vi "PupilFitEllipse.vi"(7 "Image Name":string="ellipse2", 8 "CR Ellipse":T2 {"Minor Axis"."Point 2"."Y" format="%.2f"; "Minor Axis"."Point 2"."X" format="%.2f"; "Minor Axis"."Point 1"."Y" format="%.2f"; "Minor Axis"."Point 1"."X" format="%.2f"; "Major Axis"."Point 2"."Y" format="%.2f"; "Major Axis"."Point 2"."X" format="%.2f"; "Major Axis"."Point 1"."Y" format="%.2f"; "Major Axis"."Point 1"."X" format="%.2f"; "Center"."Y" format="%.2f"; "Center"."X" format="%.2f"}, 9 "r":dbl=100.0, 10 "rough center":cluster{"Pos. X":i32, "Pos. Y":i32}, 11 "Image Src":T3) -> (0 "输出簇":T1, 1 "Image Out":T3, 2 "Valid Fit":bool, 3 "Ellipse 2":T2 {"Minor Axis"."Point 2"."Y" format="%.2f"; "Minor Axis"."Point 2"."X" format="%.2f"; "Minor Axis"."Point 1"."Y" format="%.2f"; "Minor Axis"."Point 1"."X" format="%.2f"; "Major Axis"."Point 2"."Y" format="%.2f"; "Major Axis"."Point 2"."X" format="%.2f"; "Major Axis"."Point 1"."Y" format="%.2f"; "Major Axis"."Point 1"."X" format="%.2f"; "Center"."Y" format="%.2f"; "Center"."X" format="%.2f"})   [LabVIEW 2011]
uses:
  <vilib>/vision/Image Controls.llb/IMAQ Image.ctl
  <vilib>/vision/NI_Vision_Development_Module.lvlib
panel:
  out "数值":i32
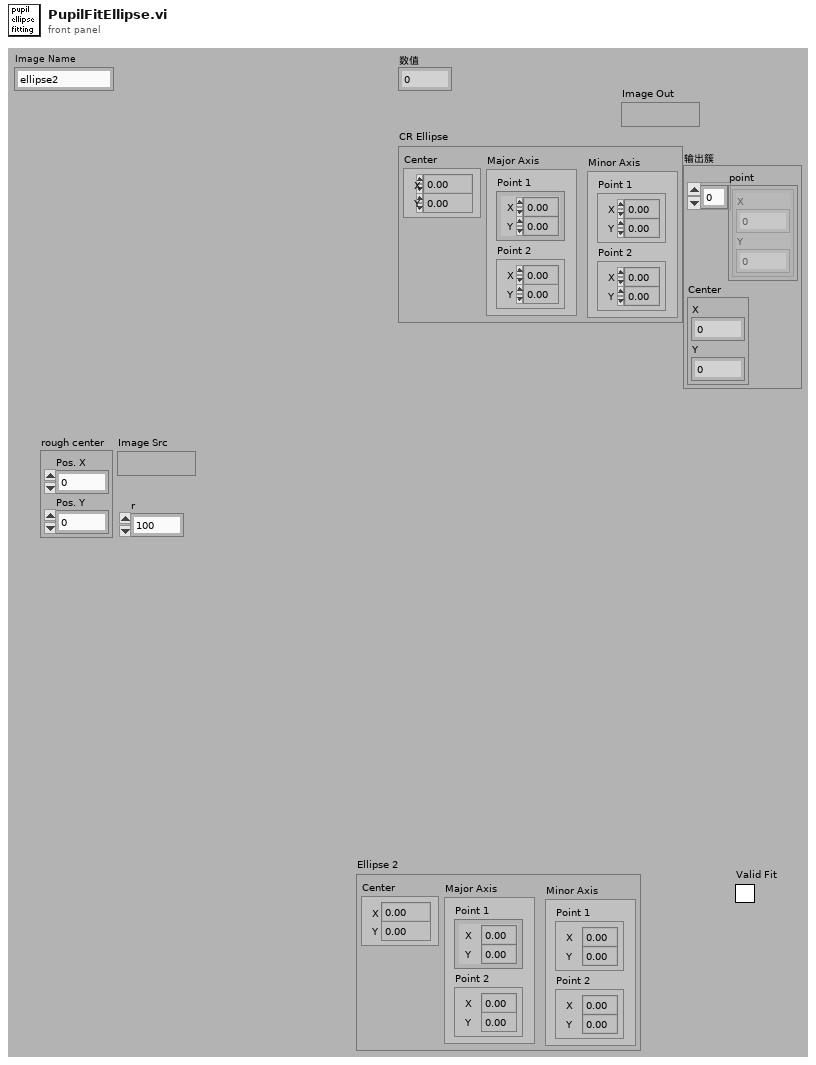
[diagram p1: front panel]
types:
  T1 = cluster{"point":cluster{"X":i32, "Y":i32}[], "Center":cluster{"X":sgl, "Y":sgl}}
  T2 = cluster{"Center":cluster{"X":sgl, "Y":sgl}, "Major Axis":cluster{"Point 1":cluster{"X":sgl, "Y":sgl}, "Point 2":cluster{"X":sgl, "Y":sgl}}, "Minor Axis":cluster{"Point 1":cluster{"X":sgl, "Y":sgl}, "Point 2":cluster{"X":sgl, "Y":sgl}}}
  T3 = typedef "IMAQ Image.ctl" = refnum<image>
  T4 = enum32{"Differentiation", "Gradient", "Prewitt", "Roberts", "Sigma", "Sobel"}
  T5 = typedef "Image Type" = u32
  T6 = cluster{"Point 1":cluster{"X":sgl, "Y":sgl}, "Point 2":cluster{"X":sgl, "Y":sgl}}
  T7 = cluster{cluster{"X":i32, "Y":i32}[], "Center":cluster{"X":sgl, "Y":sgl}}
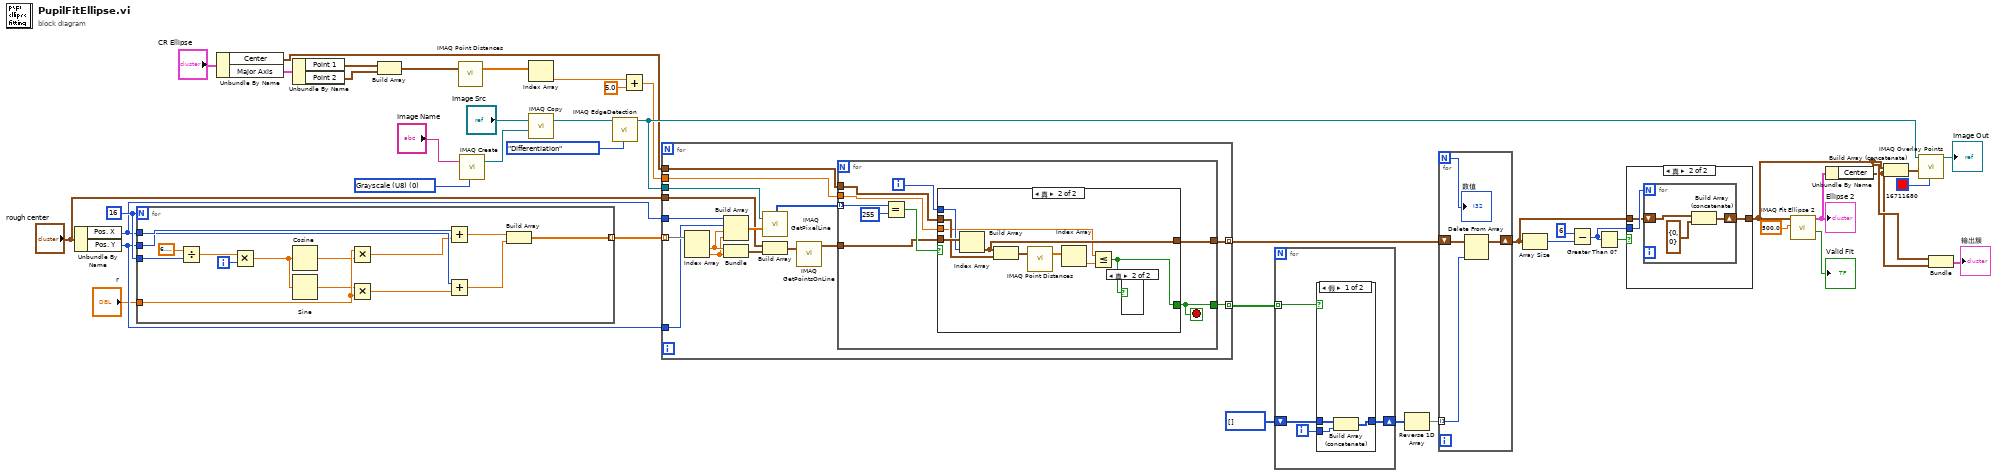
[diagram p0: block diagram]
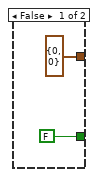
[diagram p4: hidden frame]
diagram:
  w8 = 16
  w42 = T5 0 items=["Grayscale (U8)", "Grayscale (I16)", "Grayscale (SGL)", "Complex (CSG)", "RGB (U32)", "HSL (U32)", "RGB (U64)", "Grayscale (U16)"] ("Image Type")
  n1 = Unbundle By Name("rough center") -> ("Pos. X"=w7:i32, "Pos. Y"=w6:i32)
  n2 = for {
    N: w8 -> [_]
    tunnel: w8 -> [w57]
    tunnel: [w53] -> w4 mode=indexing
    tunnel: w7 -> [w52]
    tunnel: w6 -> [w50]
    tunnel: "r" -> [w47]
    i -> [w48]
    n3 = Divide(x=6.283185307179586, y=w57) -> (x/y=w55:dbl)
    n4 = Multiply(x=w55, y=w48) -> (x*y=w54:dbl)
    n5 = Cosine(x=w54) -> (cos(x)=w44:dbl)
    n6 = Sine(x=w54) -> (sin(x)=w46:dbl)
    n7 = Multiply(x=w47, y=w44) -> (x*y=w43:dbl)
    n8 = Multiply(x=w46, y=w47) -> (x*y=w45:dbl)
    n9 = Add(x=w52, y=w43) -> (x+y=w51:dbl)
    n10 = Add(x=w50, y=w45) -> (x+y=w49:dbl)
    n11 = Build Array(w51, w49) -> (w53:dbl[])
  }
  n12 = Unbundle By Name("CR Ellipse") -> ("Center"=w22:cluster{"X":sgl, "Y":sgl}, "Major Axis"=w27:T6)
  n13 = Unbundle By Name(w27) -> ("Point 1"=w26:cluster{"X":sgl, "Y":sgl}, "Point 2"=w25:cluster{"X":sgl, "Y":sgl})
  n14 = Build Array(w26, w25) -> (w24:cluster{"X":sgl, "Y":sgl}[])
  n15 = call "IMAQ Point Distances"("Points"=w24) -> ("Distances"=w23:sgl[])  [unwired: 1 in, 4 out]
  n16 = call "IMAQ Create"("Image Name"="Image Name", "Image Type"=w42) -> ("New Image"=w40:T3)  [unwired: 2 in, 2 out]
  n17 = Index Array(array=w23) -> (element=w10:sgl)  [unwired: 1 in]
  n18 = call "IMAQ Copy"("Image Dst"=w40, "Image Src"="Image Src") -> ("Image Dst Out"=w39:T3)  [unwired: 1 in, 4 out]
  n19 = call "IMAQ EdgeDetection"("Method"=T4."Differentiation", "Image Src"=w39) -> ("Image Dst Out"=w32:T3)  [unwired: 4 in, 5 out]
  n20 = Add(x=w10, y=sgl 5.0) -> (x+y=w9:sgl)
  n21 = for {
    tunnel: w4 -> [w73] mode=indexing
    tunnel: w7 -> [w72]
    tunnel: w6 -> [w71]
    tunnel: w32 -> [w70]
    tunnel: "rough center" -> [w65]
    tunnel: [w61] -> w17 mode=indexing
    tunnel: w22 -> [w60]
    tunnel: w9 -> [w59]
    tunnel: [w58] -> w21 mode=indexing
    n22 = Index Array(array=w73) -> (element #1=w68:dbl, element #2=w67:dbl)  [unwired: 2 in]
    n23 = Build Array(w72, w71, w68, w67) -> (w69:dbl[])
    n24 = Bundle(w68, w67) -> (w66:cluster{dbl, dbl})  [unwired: 1 out]
    n25 = call "IMAQ GetPixelLine"("Line Coordinates"=w69, "Image"=w70) -> ("Pixels Line (U8)"=w63:u8[])  [unwired: 1 in, 5 out]
    n26 = Build Array(w65, w66) -> (w64:cluster{"Pos. X":dbl, "Pos. Y":dbl}[])
    n27 = call "IMAQ GetPointsOnLine"("Endpoints"=w64) -> ("Points of the Line"=w62:cluster{"X":i32, "Y":i32}[])  [unwired: 1 in, 2 out]
    n28 = for {
      tunnel: w63 -> [w82] mode=indexing
      tunnel: w62 -> [w79]
      tunnel: [w78] -> w61
      tunnel: w60 -> [w76]
      tunnel: w59 -> [w75]
      tunnel: [w74] -> w58
      i -> [w77]
      stop <- w74 stop-if-true
      n29 = Equal?(x=w82, y=u8 255) -> (x = y?=w80:bool)
      n30 = case shown="真" w80 {
        tunnel: w79 -> [_ w93]
        tunnel: [cluster{"X":i32, "Y":i32} {"X"=0, "Y"=0} w90] -> w78
        tunnel: w77 -> [_ w92]
        tunnel: w76 -> [_ w89]
        tunnel: w75 -> [_ w86]
        tunnel: [FALSE w85] -> w74
        frame False {
        }
        frame True {
          n31 = Index Array(array=w93, index=w92) -> (element=w90:cluster{"X":i32, "Y":i32})
          n32 = Build Array(w90, w89) -> (w88:cluster{"X":sgl, "Y":sgl}[])
          n33 = call "IMAQ Point Distances"("Points"=w88) -> ("Distances"=w91:sgl[])  [unwired: 1 in, 4 out]
          n34 = Index Array(array=w91) -> (element=w87:sgl)  [unwired: 1 in]
          n35 = Less Or Equal?(x=w86, y=w87) -> (x <= y?=w85:bool)
          n36 = case shown="真" w85 {
            frame False {
            }
            frame True {
            }
          }
        }
      }
    }
  }
  n37 = for {
    tunnel: w21 -> [w97] mode=indexing
    shift-right: [w95] -> w19
    shift-left: i32[] [] -> [w94]
    i -> [w96]
    n38 = case shown="假" w97 {
      tunnel: w96 -> [w100 _]
      tunnel: [w98 w101] -> w95
      tunnel: w94 -> [w99 w101]
      frame False {
        n39 = Build Array (concatenate)(w99, w100) -> (w98:i32[])
      }
      frame True {
      }
    }
  }
  n40 = Reverse 1D Array(array=w19) -> (reversed array=w18:i32[])
  n41 = for {
    N -> [w102]
    tunnel: w18 -> [w104] mode=indexing
    shift-right: [w103] -> w12
    shift-left: w17 -> [w105]
    n42 = Delete From Array(array=w105, index=w104) -> (array with subset deleted=w103:cluster{"X":i32, "Y":i32}[])  [unwired: 1 in, 1 out]
    "数值" <- w102
  }
  n43 = Array Size(array=w12) -> (size(s)=w15:i32)
  n44 = Subtract(x=6 ("y"), y=w15) -> (x-y=w13:i32)
  n45 = Greater Than 0?(x=w13) -> (x > 0?=w14:bool)
  n46 = case shown="真" w14 {
    tunnel: w13 -> [_ w109]
    tunnel: w12 -> [w106 w108]
    tunnel: [w106 w107] -> w3
    frame False {
    }
    frame True {
      n47 = for {
        N: w109 -> [_]
        shift-right: [w110] -> w107
        shift-left: w108 -> [w112]
        n48 = Build Array (concatenate)(w112, cluster{"X":i32, "Y":i32} {"X"=0, "Y"=0}) -> (w110:cluster{"X":i32, "Y":i32}[])
      }
    }
  }
  n49 = call "IMAQ Fit Ellipse 2"("Minimum Score"=500.0, "Radial Points"=w3) -> ("Valid Fit"=→"Valid Fit":bool, "Ellipse"=w34:T2)  [unwired: 4 in, 4 out]
  "Ellipse 2" <- w34
  n50 = Unbundle By Name(w34) -> ("Center"=w2:cluster{"X":sgl, "Y":sgl})
  n51 = Build Array (concatenate)(w3, w2) -> (w33:cluster{"X":sgl, "Y":sgl}[])
  n52 = call "IMAQ Overlay Points"("Color"=u32 16711680, "Array of Points"=w33, "Image"=w32) -> ("Image Out"=→"Image Out":T3)  [unwired: 3 in, 5 out]
  n53 = Bundle(w3, "Center"=w2) -> (→"输出簇":T7)  [unwired: 1 out]
